vi "delta timevi.vi"(5 "niqiest frequecy":dbl, 7 "niqiest band":dbl, 10 "signal in 2":waveform(dbl), 11 "signal in 1":waveform(dbl)) -> (1 "PSD 1":cluster{"f0":dbl, "df":dbl, "magnitude":dbl[]} {"magnitude" format="%.2p"; "f0" format="%0.2p"; "df" format="%0.2p"}, 2 "PSD 0":cluster{"f0":dbl, "df":dbl, "magnitude":dbl[]} {"magnitude" format="%.2p"; "f0" format="%0.2p"; "df" format="%0.2p"}, 3 "d time":cluster{"frequncy":dbl, "d time":dbl}[](array[cluster]) {"frequncy" format="%#_6p"})   [LabVIEW 2021]
uses:
  <vilib>/Analysis/4window.llb/windowTd.ctl
  <vilib>/Analysis/3filter.llb/Filter Passband Type.ctl
  <vilib>/Analysis/2dsp.llb/1D Cross Correlation (CDB).vi
  <vilib>/measure/maspectr.llb/FFT Spectrum (Mag-Phase) for 1 Chan.vi
  <vilib>/Analysis/1siggen.llb/Ramp Pattern by Delta.vi
  <vilib>/Analysis/3filter.llb/Chebyshev Filter (CDB).vi
  <vilib>/measure/maspectr.llb/FFT Spectrum (Mag-Phase) for 1 Chan (CDB).vi
  <vilib>/measure/NI_MAPro.lvlib
  <vilib>/Analysis/NI_AALPro.lvlib
  <vilib>/Analysis/NI_AALBase.lvlib
  <vilib>/Analysis/3filter.llb/Chebyshev Filter (DBL).vi
  <vilib>/Analysis/NI_AAL_SigProc.lvlib
panel:
  out "after 2":waveform(dbl)(graph)
  out "PSD 0":cluster{"f0":dbl, "df":dbl, "magnitude":dbl[]}[](graph)
  out "before":waveform(dbl)(graph)
  out "after":waveform(dbl)(graph)
  out "Waveform Graph":dbl[](graph)
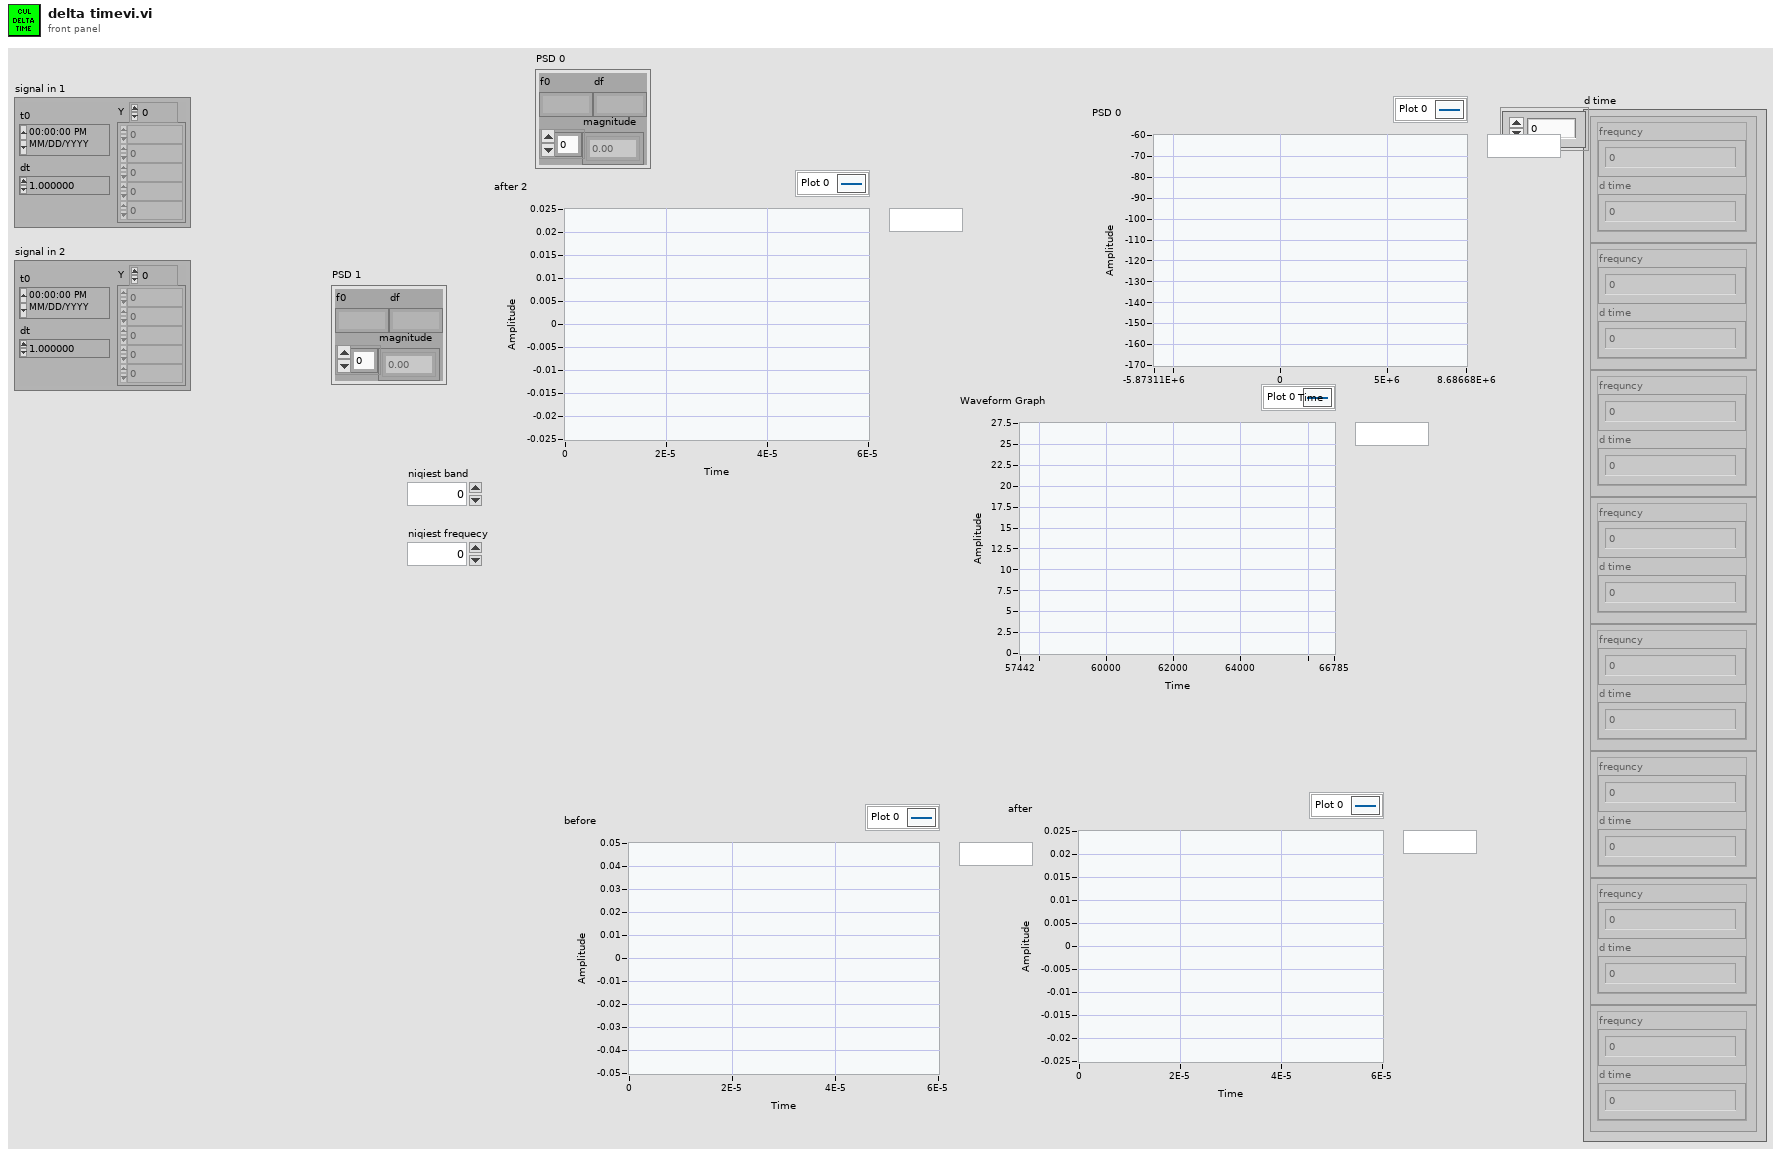
[diagram p1: front panel]
types:
  T1 = cluster{"dB On (F)":bool, "unwrap phase (F)":bool, "convert to degree (F)":bool}
  T2 = typedef "NI_AALPro.lvlib/windowTd.ctl" = u32
  T3 = typedef "NI_AALBase.lvlib/Filter Passband Type.ctl" = enum32{"Lowpass", "Highpass", "Bandpass", "Bandstop"}
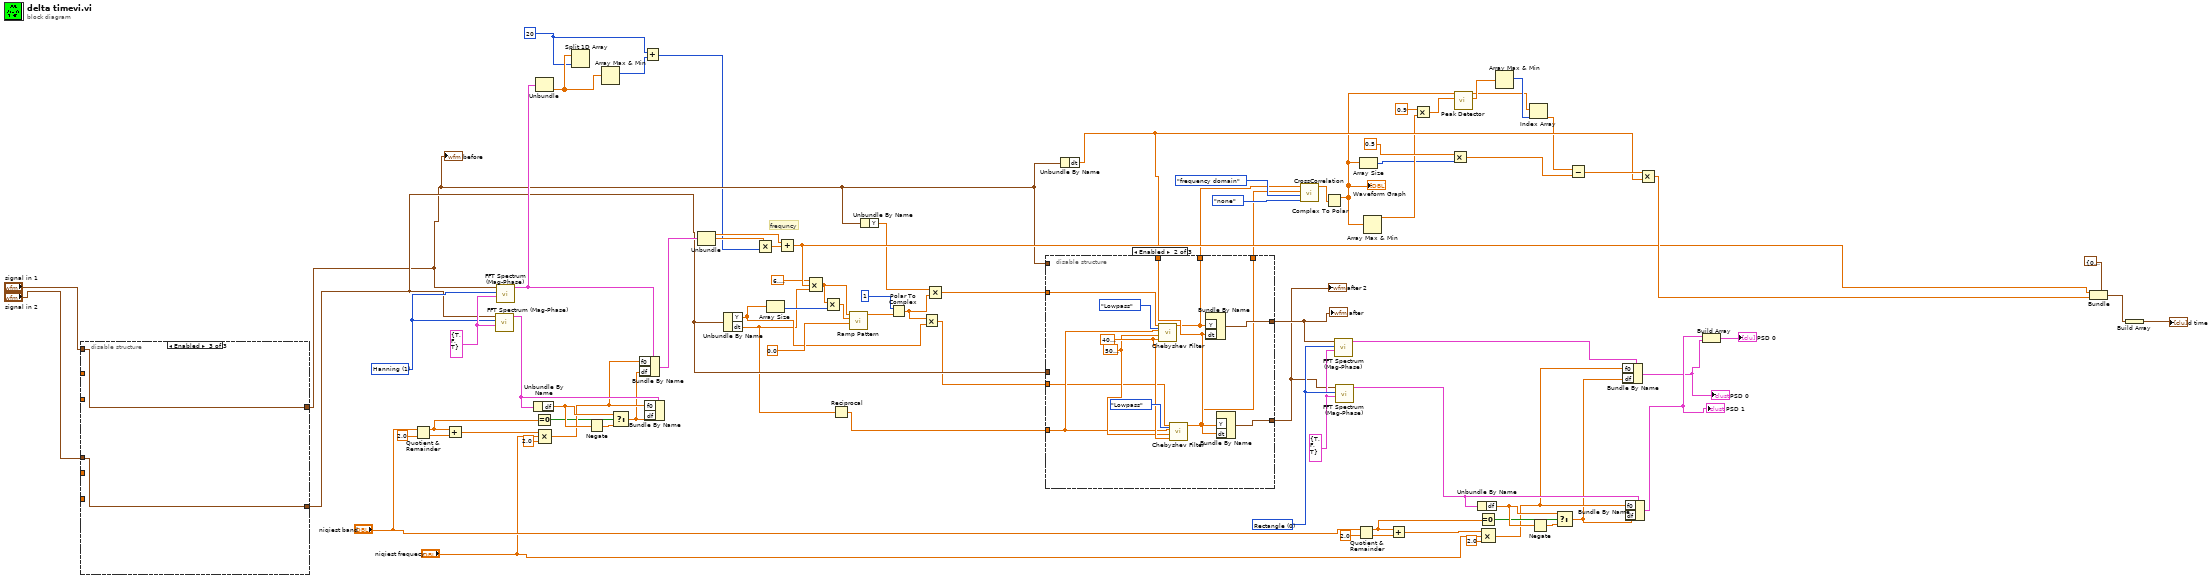
[diagram p0: block diagram]
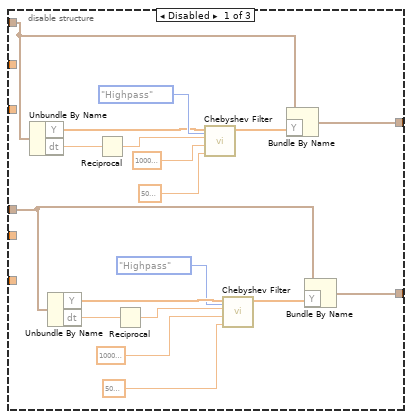
[diagram p2: hidden frame]
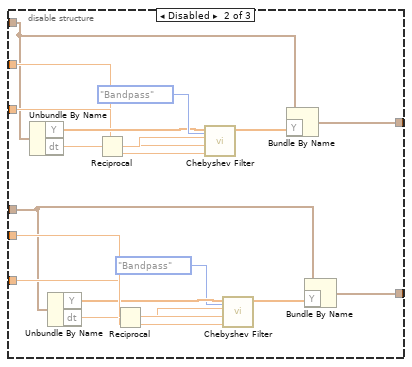
[diagram p3: hidden frame]
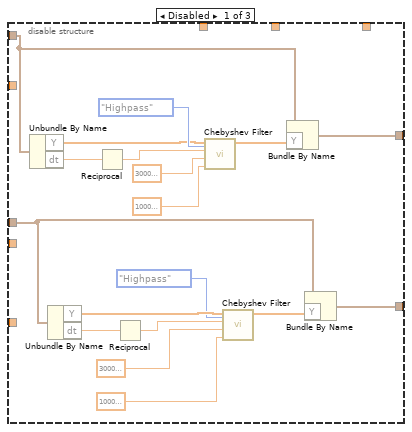
[diagram p4: hidden frame]
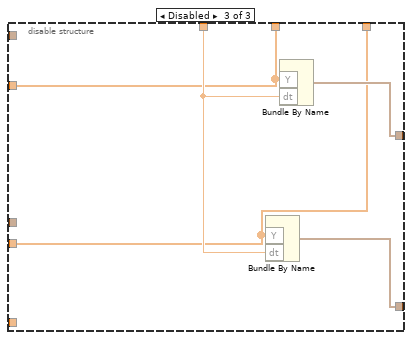
[diagram p5: hidden frame]
diagram:
  w29 = 20 ("index")
  w56 = T1 {"dB On (F)"=TRUE, "unwrap phase (F)"=FALSE, "convert to degree (F)"=TRUE} ("view")
  w57 = T2 0 items=["Rectangle"=0, "Hanning"=1, "Hamming"=2, "Blackman-Harris"=3, "Exact Blackman"=4, "Blackman"=5, "Flat Top"=6, "4 Term B-Harris "=7, "7 Term B-Harris"=8, "Low Sidelobe"=9, "Blackman Nuttall"=11, "Triangle"=30, "Bartlett-Hanning"=31, "Bohman"=32, "Parzen"=33, "Welch"=34, "Kaiser"=60, "Dolph-Chebyshev"=61, "Gaussian"=62] ("window")
  w83 = T2 1 items=["Rectangle"=0, "Hanning"=1, "Hamming"=2, "Blackman-Harris"=3, "Exact Blackman"=4, "Blackman"=5, "Flat Top"=6, "4 Term B-Harris "=7, "7 Term B-Harris"=8, "Low Sidelobe"=9, "Blackman Nuttall"=11, "Triangle"=30, "Bartlett-Hanning"=31, "Bohman"=32, "Parzen"=33, "Welch"=34, "Kaiser"=60, "Dolph-Chebyshev"=61, "Gaussian"=62] ("window")
  w84 = T1 {"dB On (F)"=TRUE, "unwrap phase (F)"=FALSE, "convert to degree (F)"=TRUE} ("view")
  # "frequncy"
  n1 = disable-structure shown="Enabled" {
    disable-tunnel: _ -> [_ w116 _]
    disable-tunnel: _ -> [_ w115 _]
    disable-tunnel: _ -> [_ w112 _]
    disable-tunnel: _ -> [_ w111 _]
    disable-tunnel: "signal in 2" -> [w92 w106 w121]
    disable-tunnel: [w85 w105 w121] -> w53
    disable-tunnel: [w91 w104 w122] -> w40
    disable-tunnel: "signal in 1" -> [w90 w103 w122]
    frame Disabled {
      n2 = Unbundle By Name(w90) -> ("Y"=w101:dbl[], "dt"=w100:dbl)
      n3 = Unbundle By Name(w92) -> ("Y"=w94:dbl[], "dt"=w95:dbl)
      n4 = Reciprocal(x=w100) -> (1/x=w99:dbl)
      n5 = Reciprocal(x=w95) -> (1/x=w96:dbl)
      n6 = call-poly <vilib>:"Chebyshev Filter.vi"("filter type"=Filter_Passband_Type."Highpass", "low cutoff freq: fl"=5000000.0 ("high cutoff freq: fh"), "high cutoff freq: fh"=10000000.0, "sampling freq: fs"=w99, "X"=w101) -> ("Filtered X"=w98:dbl[])  [unwired: 5 in, 1 out]
      n7 = call-poly <vilib>:"Chebyshev Filter.vi"("filter type"=Filter_Passband_Type."Highpass", "low cutoff freq: fl"=5000000.0 ("high cutoff freq: fh"), "high cutoff freq: fh"=10000000.0, "sampling freq: fs"=w96, "X"=w94) -> ("Filtered X"=w97:dbl[])  [unwired: 5 in, 1 out]
      n8 = Bundle By Name(cluster=w90, "Y"=w98) -> (w91:waveform(dbl))
      n9 = Bundle By Name(cluster=w92, "Y"=w97) -> (w85:waveform(dbl))
    }
    frame Disabled {
      n10 = Unbundle By Name(w103) -> ("Y"=w119:dbl[], "dt"=w118:dbl)
      n11 = Unbundle By Name(w106) -> ("Y"=w108:dbl[], "dt"=w109:dbl)
      n12 = Reciprocal(x=w118) -> (1/x=w117:dbl)
      n13 = Reciprocal(x=w109) -> (1/x=w110:dbl)
      n14 = call-poly <vilib>:"Chebyshev Filter.vi"("filter type"=Filter_Passband_Type."Bandpass", "low cutoff freq: fl"=w116, "high cutoff freq: fh"=w115, "sampling freq: fs"=w117, "X"=w119) -> ("Filtered X"=w114:dbl[])  [unwired: 5 in, 1 out]
      n15 = call-poly <vilib>:"Chebyshev Filter.vi"("filter type"=Filter_Passband_Type."Bandpass", "low cutoff freq: fl"=w111, "high cutoff freq: fh"=w112, "sampling freq: fs"=w110, "X"=w108) -> ("Filtered X"=w113:dbl[])  [unwired: 5 in, 1 out]
      n16 = Bundle By Name(cluster=w103, "Y"=w114) -> (w104:waveform(dbl))
      n17 = Bundle By Name(cluster=w106, "Y"=w113) -> (w105:waveform(dbl))
    }
    frame Enabled {
    }
  }
  "before" <- w40
  n18 = Quotient & Remainder(x="niqiest band", y=2.0) -> (x-y*floor(x/y)=w78:dbl, floor(x/y)=w80:dbl)
  n19 = Add(x=w78, y=w80) -> (x+y=w79:dbl)
  n20 = call-poly <vilib>:"FFT Spectrum (Mag-Phase).vi"("view"=w84, "window"=w83, "time signal"=w53) -> ("magnitude"=w82:cluster{"f0":dbl, "df":dbl, "magnitude":dbl[]})  [unwired: 4 in, 4 out]
  n21 = call-poly <vilib>:"FFT Spectrum (Mag-Phase).vi"("view"=w84, "window"=w83, "time signal"=w40) -> ("magnitude"=w64:cluster{"f0":dbl, "df":dbl, "magnitude":dbl[]})  [unwired: 4 in, 4 out]
  n22 = Unbundle By Name(w82) -> ("df"=w76:dbl)
  n23 = Unbundle(w64) -> ("magnitude"=w31:dbl[])  [unwired: 2 out]
  n24 = Equal To 0?(x=w78) -> (x = 0?=w72:bool)
  n25 = Compound Arithmetic op=MULTIPLY(w79, "niqiest frequecy", 2.0 ("value")) -> (w75:dbl)
  n26 = Split 1D Array(array=w31, index=w29) -> ()  [unwired: 2 out]
  n27 = Negate(x=w76) -> (-x=w77:dbl)
  n28 = Array Max & Min(array=w31) -> (max index (indices)=w30:i32)  [unwired: 3 out]
  n29 = Select(t=w76, s=w72, f=w77) -> (s? t:f=w74:dbl)
  n30 = Bundle By Name(cluster=w64, "f0"=w75, "df"=w74) -> (w58:cluster{"f0":dbl, "df":dbl, "magnitude":dbl[]})
  n31 = Add(x=w29, y=w30) -> (x+y=w28:i32)
  n32 = Bundle By Name(cluster=w82, "f0"=w75, "df"=w74) -> ()  [unwired: 1 out]
  n33 = Unbundle(w58) -> ("f0"=w66:dbl, "df"=w65:dbl)  [unwired: 1 out]
  n34 = Unbundle By Name(w53) -> ("Y"=w44:dbl[], "dt"=w43:dbl)
  n35 = Multiply(x=w65, y=w28) -> (x*y=w67:dbl)
  n36 = Array Size(array=w44) -> (size(s)=w48:i32)
  n37 = Add(x=w66, y=w67) -> (x+y=w51:dbl)
  n38 = Compound Arithmetic op=MULTIPLY(6.283185307179586, w51, w43) -> (w49:dbl)
  n39 = Multiply(x=w49, y=w48) -> (x*y=w47:dbl)
  n40 = Reciprocal(x=w43) -> (1/x=w42:dbl)
  n41 = call-poly <vilib>:"Ramp Pattern.vi"("start"=0.0, "end"=w47, "delta"=w49) -> ("Ramp Pattern"=w46:dbl[])  [unwired: 6 in, 2 out]
  n42 = Unbundle By Name(w40) -> ("Y"=w38:dbl[])
  n43 = Polar To Complex(1:w46, 2:1) -> (0:w39:cdb[])
  n44 = Multiply(x=w39, y=w44) -> (x*y=w41:cdb[])
  n45 = Multiply(x=w38, y=w39) -> (x*y=w37:cdb[])
  n46 = Unbundle By Name(w40) -> ("dt"=w36:dbl)
  n47 = disable-structure shown="Enabled" {
    disable-tunnel: w53 -> [w130 _ _]
    disable-tunnel: [w129 w150 w156] -> w32
    disable-tunnel: [w128 w149 w155] -> w35
    disable-tunnel: w40 -> [w127 _ _]
    disable-tunnel: w42 -> [_ w146 _]
    disable-tunnel: w41 -> [_ w145 w153]
    disable-tunnel: w37 -> [_ w144 w154]
    disable-tunnel: w36 -> [_ w143 w157]
    disable-tunnel: [_ w142 w154] -> w27
    disable-tunnel: [_ w141 w153] -> w26
    frame Disabled {
      n48 = Unbundle By Name(w127) -> ("Y"=w139:dbl[], "dt"=w138:dbl)
      n49 = Unbundle By Name(w130) -> ("Y"=w132:dbl[], "dt"=w133:dbl)
      n50 = Reciprocal(x=w138) -> (1/x=w137:dbl)
      n51 = Reciprocal(x=w133) -> (1/x=w134:dbl)
      n52 = call-poly <vilib>:"Chebyshev Filter.vi"("filter type"=Filter_Passband_Type."Highpass", "low cutoff freq: fl"=10000000.0 ("high cutoff freq: fh"), "high cutoff freq: fh"=30000000.0, "sampling freq: fs"=w137, "X"=w139) -> ("Filtered X"=w136:dbl[])  [unwired: 5 in, 1 out]
      n53 = call-poly <vilib>:"Chebyshev Filter.vi"("filter type"=Filter_Passband_Type."Highpass", "low cutoff freq: fl"=10000000.0 ("high cutoff freq: fh"), "high cutoff freq: fh"=30000000.0, "sampling freq: fs"=w134, "X"=w132) -> ("Filtered X"=w135:dbl[])  [unwired: 5 in, 1 out]
      n54 = Bundle By Name(cluster=w127, "Y"=w136) -> (w128:waveform(dbl))
      n55 = Bundle By Name(cluster=w130, "Y"=w135) -> (w129:waveform(dbl))
    }
    frame Enabled {
      w147 = 5000000.0 ("y")
      w148 = 4000000.0 ("y")
      n56 = call-poly <vilib>:"Chebyshev Filter.vi"("filter type"=Filter_Passband_Type."Lowpass", "low cutoff freq: fl"=w148, "high cutoff freq: fh"=w147, "sampling freq: fs"=w146, "X"=w144) -> ("Filtered X"=w142:cdb[])  [unwired: 5 in, 1 out]
      n57 = call-poly <vilib>:"Chebyshev Filter.vi"("filter type"=Filter_Passband_Type."Lowpass", "low cutoff freq: fl"=w148, "high cutoff freq: fh"=w147, "sampling freq: fs"=w146, "X"=w145) -> ("Filtered X"=w141:cdb[])  [unwired: 5 in, 1 out]
      n58 = Bundle By Name("Y"=w142, "dt"=w143) -> (w149:waveform(cdb))  [unwired: 1 in]
      n59 = Bundle By Name("Y"=w141, "dt"=w143) -> (w150:waveform(cdb))  [unwired: 1 in]
    }
    frame Disabled {
      n60 = Bundle By Name("Y"=w153, "dt"=w157) -> (w156:waveform(cdb))  [unwired: 1 in]
      n61 = Bundle By Name("Y"=w154, "dt"=w157) -> (w155:waveform(cdb))  [unwired: 1 in]
    }
  }
  "after" <- w35
  "after 2" <- w32
  n62 = call-poly <vilib>:"CrossCorrelation.vi"("normalization"=enum32{"none", "unbiased", "biased"}."none", "algorithm"=enum32{"direct", "frequency domain"}."frequency domain", "Y"=w26, "X"=w27) -> ("Rxy"=w34:cdb[])  [unwired: 6 in, 1 out]
  n63 = Complex To Polar(r * e^(i*theta)=w34) -> (r=w25:dbl[])  [unwired: 1 out]
  "Waveform Graph" <- w25
  n64 = call-poly <vilib>:"FFT Spectrum (Mag-Phase).vi"("view"=w56, "window"=w57, "time signal"=w35) -> ("magnitude"=w7:cluster{"f0":dbl, "df":dbl, "magnitude":dbl[]})  [unwired: 4 in, 4 out]
  n65 = call-poly <vilib>:"FFT Spectrum (Mag-Phase).vi"("view"=w56, "window"=w57, "time signal"=w32) -> ("magnitude"=w9:cluster{"f0":dbl, "df":dbl, "magnitude":dbl[]})  [unwired: 4 in, 4 out]
  n66 = Quotient & Remainder(x="niqiest band", y=2.0) -> (x-y*floor(x/y)=w14:dbl, floor(x/y)=w16:dbl)
  n67 = Array Size(array=w25) -> (size(s)=w1:i32)
  n68 = Array Max & Min(array=w25) -> (max value=w24:dbl)  [unwired: 3 out]
  n69 = Add(x=w14, y=w16) -> (x+y=w15:dbl)
  n70 = Multiply(x=0.9, y=w24) -> (x*y=w22:dbl)
  n71 = Multiply(x=0.5 ("y"), y=w1) -> (x*y=w70:dbl)
  n72 = call <vilib>:"Peak Detector.vi"("threshold"=w22, "X"=w25) -> ("Amplitudes"=w21:dbl[], "Locations"=w19:dbl[])  [unwired: 5 in, 3 out]
  n73 = Unbundle By Name(w9) -> ("df"=w12:dbl)
  n74 = Equal To 0?(x=w14) -> (x = 0?=w10:bool)
  n75 = Compound Arithmetic op=MULTIPLY(w15, "niqiest frequecy", 2.0 ("value")) -> (w6:dbl)
  n76 = Array Max & Min(array=w21) -> (max index (indices)=w20:i32)  [unwired: 3 out]
  n77 = Index Array(array=w19, index=w20) -> (element=w18:dbl)
  n78 = Negate(x=w12) -> (-x=w13:dbl)
  n79 = Select(t=w12, s=w10, f=w13) -> (s? t:f=w5:dbl)
  n80 = Subtract(x=w18, y=w70) -> (x-y=w69:dbl)
  n81 = Bundle By Name(cluster=w7, "f0"=w6, "df"=w5) -> (w4:cluster{"f0":dbl, "df":dbl, "magnitude":dbl[]})
  "PSD 0" <- w4
  n82 = Bundle By Name(cluster=w9, "f0"=w6, "df"=w5) -> (w8:cluster{"f0":dbl, "df":dbl, "magnitude":dbl[]})
  "PSD 1" <- w8
  n83 = Multiply(x=w69, y=w36) -> (x*y=w68:dbl)
  n84 = Build Array(w8, w4) -> (→"PSD 0":cluster{"f0":dbl, "df":dbl, "magnitude":dbl[]}[])
  n85 = Bundle(cluster=cluster{"frequncy":dbl, "d time":dbl} {"frequncy"=0.0, "d time"=0.0}, "frequncy"=w51, "d time"=w68) -> (w62:cluster{"frequncy":dbl, "d time":dbl})
  n86 = Build Array(w62) -> (→"d time":cluster{"frequncy":dbl, "d time":dbl}[])
